vi "Test_AO_6711_Standalone_SubVIs.vi"(8 "error in (no error)":errorcluster, 11 "Use Software Trigger":bool=TRUE) -> (0 "error out":errorcluster)   [LabVIEW 2018]
doc: "This VI inits a waveform generation session for AWG-5421. This is a basic example that shows how to setup the board in order to generate waveforms according to a script. \nBy default this configuration uses one channel CH0, and one script trigger ScriptTrigger0. The ScriptTrigger0 is waiting for an external trigger : i.e. a digital Edge on pin PFI 0 by default.\n\nThere are various options for the script to be used. Consult the Script control help for more information on configuring the example for specific scripts."
uses:
  controls/SOFTWARE_Inputs.ctl
  controls/TRAPPING_Inputs.ctl
  controls/AO_6711_Inputs.ctl
panel:
  in  "AO 6711 Inputs":T1={"Physical Channels"="AO_6711/ao0:3", "Min Voltage"=-10.0, "Max Voltage"=10.0, "Trigger Source"="/AO_6711/PFI3", "Counter"="AO_6711/ctr0"} {"Max Voltage" min=-10.0 max=10.0; "Min Voltage" min=-10.0 max=10.0}
  out "number of samples written per channel":u32 caption="nombre d'échantillons écrits par voie"
  out "number of samples":i32
  in  "TRAPPING Inputs":T2={"Number of Channels"=4, "Init Values"=[2.0, 9.0, 9.0, 2.0], "Opening Values"=[0.0, 0.0, 0.0, 0.0], "Trapping Values"=[2.0, 9.0, 9.0, 2.0], "Emptying Values"=[-10.0, -10.0, -10.0, -10.0], "Adiabatic ON"=FALSE, "Adiabatic Duration"=0, "Adiabatic Waveforms"=["Adiabatic_None_2_2_2000", "Adiabatic_Ramp_5_0_2000", "Adiabatic_DoubleRamp_5_0_2000", "Adiabatic_RC_2_0_2000"], "Ions Accumulation ON"=FALSE, "Number of Ions Refills"=1, "Ions Opening Values"=[0.0, 0.0, 0.0, 0.0], "Ions Trapping Values"=[2.0, 9.0, 2.0, 9.0]} {"Number of Ions Refills" min=1 max=1000; "Ions Opening Values" min=-10.0 max=10.0; "Ions Trapping Values" min=-10.0 max=10.0; "Trapping Values" min=-10.0 max=10.0; "Init Values" min=-10.0 max=10.0; "Emptying Values" min=-10.0 max=10.0; "Opening Values" min=-10.0 max=10.0}
  in  "SOFTWARE Inputs":T3={"Application Directory"=path "D:/S.O.F.T.S/LABVIEW/PIL", "Software Version"="1.0.0", "Data Path"=path "D:/PIRENEA/DATA", "XML Path"=path "D:/PIRENEA/DATA", "XML File Filter"="*.xml", "XML Saved Path"=path "D:/S.O.F.T.S/LABVIEW/PIL/resources", "Excit Scripts Path"=path "D:/PIRENEA/EXCIT_SCRIPTS", "Excit Scripts File Filter"="*.txt", "Excit Waveforms Path"=path "D:/PIRENEA/EXCIT_WFMS", "Excit Waveforms File Filter"="*.bin", "Timing Scripts Path"=path "D:/PIRENEA/TIMING_SCRIPTS", "Timing Scripts File Filter"="*.txt", "Timing Waveforms Path"=path "D:/PIRENEA/TIMING_WFMS", "Timing Waveforms File Filter"="*.bin", "Trapping Waveforms Path"=path "D:/PIRENEA/TRAPPING_WFMS", "Trapping Waveforms File Filter"="*.bin"}
  # "GO_out"
  # "Gout"
  # "GI_in"
  # "Gin"
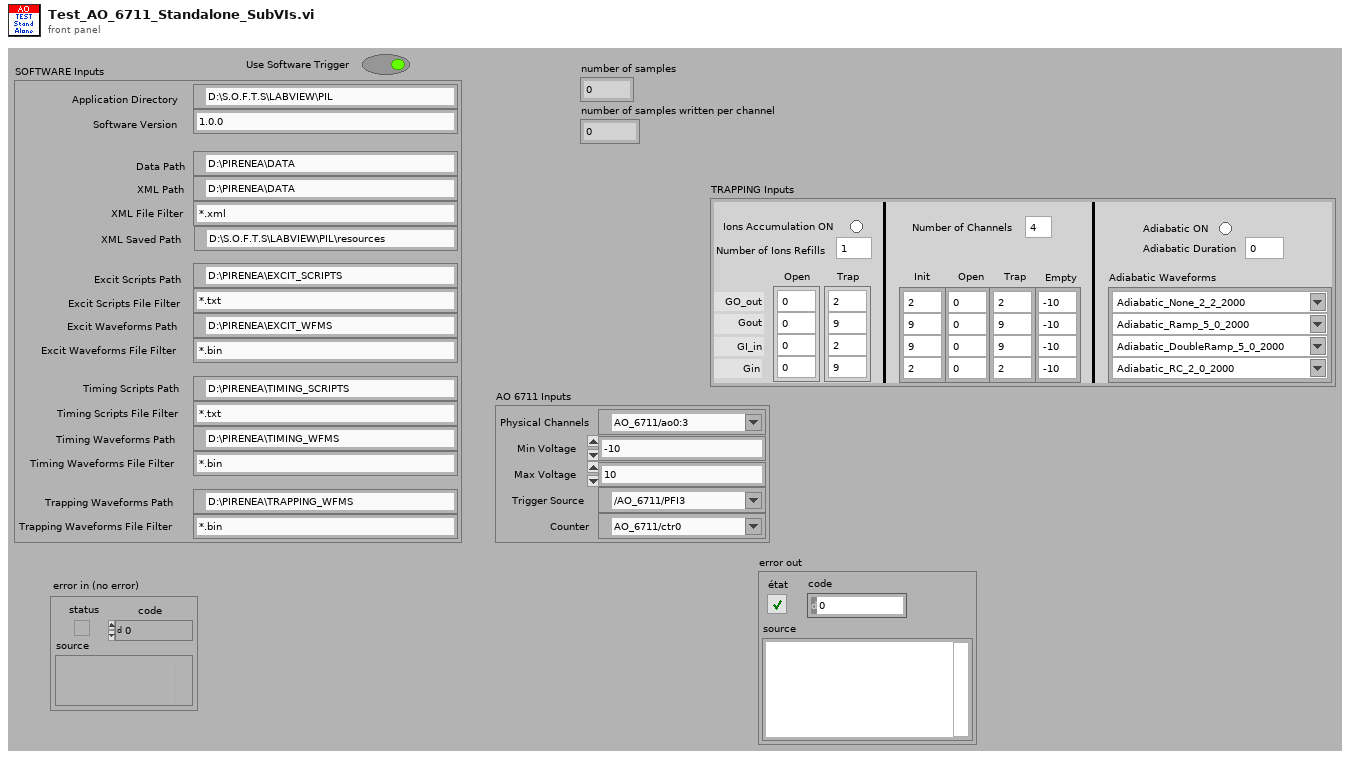
[diagram p1: front panel]
types:
  T1 = typedef "AO_6711_Inputs.ctl" = cluster{"Physical Channels":tag, "Min Voltage":dbl, "Max Voltage":dbl, "Trigger Source":tag, "Counter":tag}
  T2 = typedef "TRAPPING_Inputs.ctl" = cluster{"Number of Channels":i32, "Init Values":dbl[], "Opening Values":dbl[], "Trapping Values":dbl[], "Emptying Values":dbl[], "Adiabatic ON":bool, "Adiabatic Duration":i32, "Adiabatic Waveforms":string[], "Ions Accumulation ON":bool, "Number of Ions Refills":i32, "Ions Opening Values":dbl[], "Ions Trapping Values":dbl[]}
  T3 = typedef "SOFTWARE_Inputs.ctl" = cluster{"Application Directory":path, "Software Version":string, "Data Path":path, "XML Path":path, "XML File Filter":string, "XML Saved Path":path, "Excit Scripts Path":path, "Excit Scripts File Filter":string, "Excit Waveforms Path":path, "Excit Waveforms File Filter":string, "Timing Scripts Path":path, "Timing Scripts File Filter":string, "Timing Waveforms Path":path, "Timing Waveforms File Filter":string, "Trapping Waveforms Path":path, "Trapping Waveforms File Filter":string}
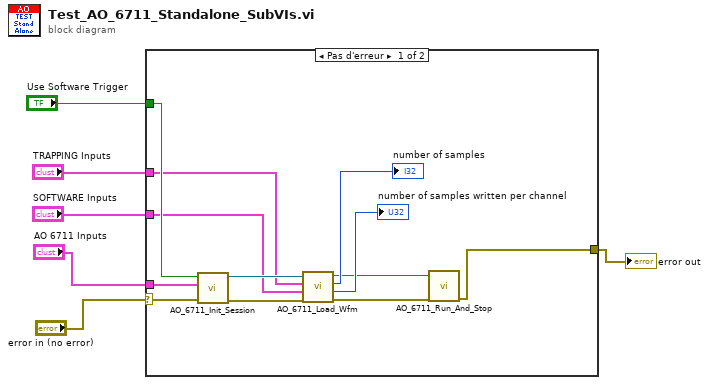
[diagram p0: block diagram]
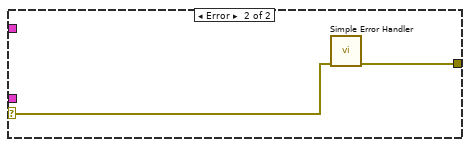
[diagram p2: hidden frame]
diagram:
  n1 = case shown="Pas d'erreur" "error in (no error)" {
    selector: "error in (no error)" -> [w18 w20]
    tunnel: [w11 w19] -> w6
    tunnel: "Use Software Trigger" -> [w16 _]
    tunnel: "SOFTWARE Inputs" -> [w15 _]
    tunnel: "TRAPPING Inputs" -> [w14 _]
    tunnel: "AO 6711 Inputs" -> [w8 _]
    frame No Error {
      n2 = call "AO_6711_Init_Session.vi"("error in (no error)"=w18, "AO 6711 Inputs"=w8, "Use Software Trigger"=w16) -> ("error out"=w13:errorcluster, "Instrument handle out"=w17:refnum<k21>)  [unwired: 7 in]
      n3 = call "AO_6711_Load_Wfm.vi"("error in (no error)"=w13, "SOFTWARE Inputs"=w15, "TRAPPING Inputs"=w14, "Instrument handle in"=w17) -> ("error out"=w12:errorcluster, "number of samples written per channel"=→"number of samples written per channel":u32, "number of samples"=→"number of samples":i32, "Instrument handle out"=w7:refnum<k21>)  [unwired: 4 in]
      n4 = call "AO_6711_Run_And_Stop.vi"("error  in"=w12, "Instrument handle in"=w7) -> ("error out"=w11:errorcluster)  [unwired: 9 in]
    }
    frame Error {
      n5 = call <vilib>:"Simple Error Handler.vi"("error in (no error)"=w20) -> ("error out"=w19:errorcluster)  [unwired: 4 in, 4 out]
    }
  }
  "error out" <- w6
